vi "Test set frequency and power.vi"() -> ()   [LabVIEW 2020, in "Harmonics.lvclass"]
uses:
  Harmonics.lvclass
  Instruments/Signal Generator/Signal Generator.lvclass
  Harmonics.lvclass/Harmonics.ctl
panel:
  out "Power":bool[](array[boolean])
  out "Freq":bool[](array[boolean])
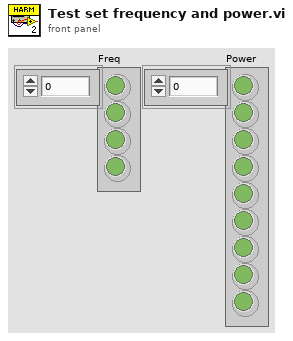
[diagram p1: front panel]
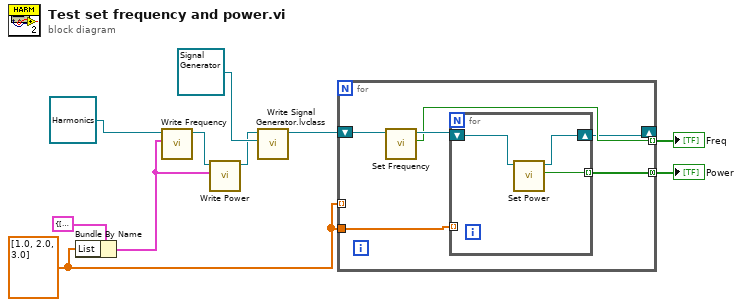
[diagram p0: block diagram]
diagram:
  w5 = dbl[] [1.0, 2.0, 3.0] ("List")
  n1 = Bundle By Name(cluster=cluster{"List":dbl[], "Index":i32, "Last":bool} {"List"=[], "Index"=0, "Last"=FALSE} ("Frequency"), "List"=w5) -> (w1:cluster{"List":dbl[], "Index":i32, "Last":bool})
  n2 = call "Write Frequency.vi"("Frequency"=w1, "Harmonics in"=refnum<class "Harmonics.lvclass"> refnum ("Harmonics.lvclass")) -> ("Harmonics out"=w3:refnum<class "Harmonics.lvclass">)  [unwired: 9 in]
  n3 = call "Write Power.vi"("Power"=w1, "Harmonics in"=w3) -> ("Harmonics out"=w2:refnum<class "Harmonics.lvclass">)  [unwired: 9 in]
  n4 = call "Write Signal Generator.lvclass.vi"("Signal Generator.lvclass"=refnum<class "Signal Generator.lvclass"> refnum, "Harmonics in"=w2) -> ("Harmonics out"=w7:refnum<class "Harmonics.lvclass">)  [unwired: 9 in]
  n5 = for {
    tunnel: [w13] -> w8 mode=indexing
    shift-right: [w11] -> _
    shift-left: w7 -> [w16]
    tunnel: w5 -> [_] mode=indexing
    tunnel: w5 -> [w15]
    tunnel: [w12] -> w4 mode=concatenating
    n6 = call "Set Frequency.vi"("Harmonics in"=w16) -> ("Last Frequency?"=w13:bool, "Harmonics out"=w14:refnum<class "Harmonics.lvclass">)  [unwired: 7 in, 2 out]
    n7 = for {
      tunnel: w15 -> [_] mode=indexing
      shift-right: [w18] -> w11
      shift-left: w14 -> [w19]
      tunnel: [w17] -> w12 mode=indexing
      n8 = call "Set Power.vi"("Harmonics in"=w19) -> ("Last Power?"=w17:bool, "Harmonics out"=w18:refnum<class "Harmonics.lvclass">)  [unwired: 7 in, 2 out]
    }
  }
  "Freq" <- w8
  "Power" <- w4
